vi "5_Sum1toNmultiples.vi"() -> ()   [LabVIEW 2015]
panel:
  out "Sum of 1 to N for multiples of 3 & 5":u32
  in  "Enter a number":u32
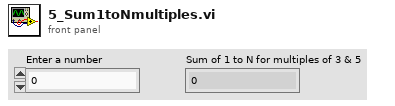
[diagram p1: front panel]
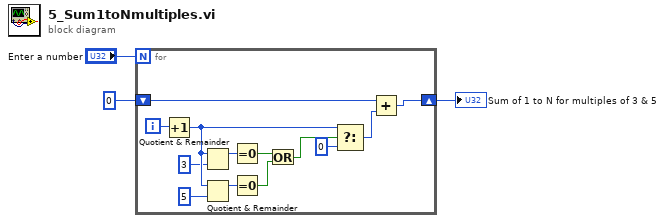
[diagram p0: block diagram]
diagram:
  n1 = for {
    N: "Enter a number" -> [_]
    shift-right: [w14] -> w1
    shift-left: 0 -> [w15]
    i -> [w16]
    n2 = Increment(x=w16) -> (x+1=w11:i32)
    n3 = Quotient & Remainder(x=w11, y=3) -> (x-y*floor(x/y)=w8:i32)  [unwired: 1 out]
    n4 = Quotient & Remainder(x=w11, y=5) -> (x-y*floor(x/y)=w7:i32)  [unwired: 1 out]
    n5 = Equal To 0?(x=w8) -> (x = 0?=w6:bool)
    n6 = Equal To 0?(x=w7) -> (x = 0?=w5:bool)
    n7 = Or(x=w6, y=w5) -> (x .or. y?=w4:bool)
    n8 = Select(t=w11, s=w4, f=0) -> (s? t:f=w13:i32)
    n9 = Add(x=w15, y=w13) -> (x+y=w14:i32)
  }
  "Sum of 1 to N for multiples of 3 & 5" <- w1
